vi "Execute.vi"(0 "reference in":refnum<class "ViPER.lvclass">, 1 "cmd":string, 2 "controls":string[](array[string]), 3 "indicators":string[](array[string]), 4 "control data":variant[](array[variant]), 5 "error in (no error)":errorcluster, 6 "must_exist":bool=TRUE, 7 "options":i32 format="%.0x", 9 "wait until done (T)":bool=TRUE) -> (14 "reference out":refnum<class "ViPER.lvclass">, 15 "exists":bool, 16 "vi reference":refnum<vi>, 18 "indicator data":variant[](array[variant]), 19 "error out":errorcluster)   [LabVIEW 2022 SP3, in "ViPER.lvlib" / "ViPER.lvclass"]
doc: "### BSD License (http://www.opensource.org/licenses/bsd-license.php) Begin ###\n\nCopyright (c) 2018 Kurt Friday www.medulla.net\n\nAll rights reserved.\n\nRedistribution and use in source and binary forms, with or without\nmodification, are permitted provided that the following conditions are met:\n\n * Redistributions of source code must retain the above copyright\n notice, this list of conditions and the following disclaimer.\n\n * Redistributions in binary form must reproduce the above copyright\n notice, this list of conditions and the following disclaimer in the\n documentation and/or other materials provided with the distribution.\n\n * Neither the name of the <organization> nor the\n names of its contributors may be used to endorse or promote products\n derived from this software without specific prior written permission.\n\nTHIS SOFTWARE IS PROVIDED BY THE COPYRIGHT HOLDERS AND CONTRIBUTORS \"AS IS\" AND\nANY EXPRESS OR IMPLIED WARRANTIES, INCLUDING, BUT NOT LIMITED TO, THE IMPLIED\nWARRANTIES OF MERCHANTABILITY AND FITNESS FOR A PARTICULAR PURPOSE ARE\nDISCLAIMED. IN NO EVENT SHALL <COPYRIGHT HOLDER> BE LIABLE FOR ANY\nDIRECT, INDIRECT, INCIDENTAL, SPECIAL, EXEMPLARY, OR CONSEQUENTIAL DAMAGES\n(INCLUDING, BUT NOT LIMITED TO, PROCUREMENT OF SUBSTITUTE GOODS OR SERVICES;\nLOSS OF USE, DATA, OR PROFITS; OR BUSINESS INTERRUPTION) HOWEVER CAUSED AND\nON ANY THEORY OF LIABILITY, WHETHER IN CONTRACT, STRICT LIABILITY, OR TORT\n(INCLUDING NEGLIGENCE OR OTHERWISE) ARISING IN ANY WAY OUT OF THE USE OF THIS\nSOFTWARE, EVEN IF ADVISED OF THE POSSIBILITY OF SUCH DAMAGE."
uses:
  ViPER.lvclass
panel:
  # "### BSD License (http://www.opensource.org/licenses/bsd-license.php) Begin ###\n\nCopyright (c) 2018  Kurt Friday www.medulla.net\n\nAll rights reserved.\n\nRedistribution and use in source and binary forms, with or without\nmodification, are permitted provided that the following conditions are met:\n\n    * Redistributions of source code must retain the above copyright\n      notice, this list of conditions and the following disclaimer.\n\n    * Redistributions in binary form must reproduce the above copyright\n      notice, this list of conditions and the following disclaimer in the\n      documentation and/or other materials provided with the distribution.\n\n    * Neither the name of the <organization> nor the\n      names of its contributors may be used to endorse or promote products\n      derived from this software without specific prior written permission.\n\nTHIS SOFTWARE IS PROVIDED BY THE COPYRIGHT HOLDERS AND CONTRIBUTORS \"AS IS\" AND\nANY EXPRESS OR IMPLIED WARRANTIES, INCLUDING, BUT NOT LIMITED TO, THE IMPLIED\nWARRANTIES OF MERCHANTABILITY AND FITNESS FOR A PARTICULAR PURPOSE ARE\nDISCLAIMED. IN NO EVENT SHALL <COPYRIGHT HOLDER> BE LIABLE FOR ANY\nDIRECT, INDIRECT, INCIDENTAL, SPECIAL, EXEMPLARY, OR CONSEQUENTIAL DAMAGES\n(INCLUDING, BUT NOT LIMITED TO, PROCUREMENT OF SUBSTITUTE GOODS OR SERVICES;\nLOSS OF USE, DATA, OR PROFITS; OR BUSINESS INTERRUPTION) HOWEVER CAUSED AND\nON ANY THEORY OF LIABILITY, WHETHER IN CONTRACT, STRICT LIABILITY, OR TORT\n(INCLUDING NEGLIGENCE OR OTHERWISE) ARISING IN ANY WAY OUT OF THE USE OF THIS\nSOFTWARE, EVEN IF ADVISED OF THE POSSIBILITY OF SUCH DAMAGE."
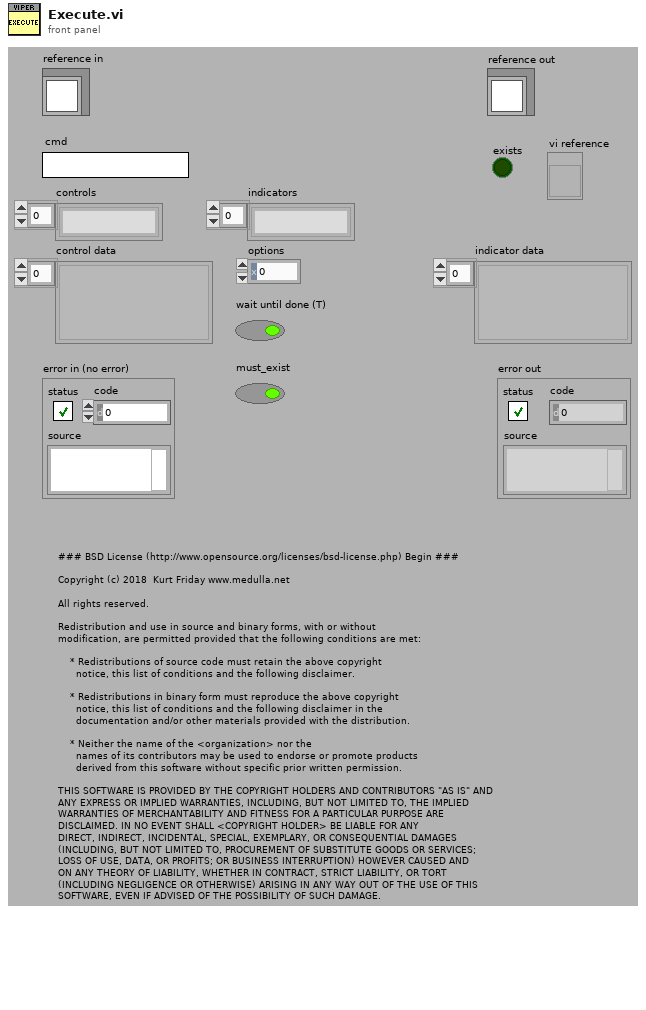
[diagram p1: front panel]
types:
  T1 = typedef "ViPER.lvlib/ViPER.lvclass/ObjectAttributes.ctl" = cluster{"Object":T2, "Ancestors":T4[], "Config":T5, "Init_OK":bool, "Hierachy":string[], "PPL?":bool[], "SFP_Open":bool[], "Config_SFP_Open":bool[], "SoftFP_event":refnum<user-event>[], "ConfigFP_event":refnum<user-event>[], "SoftFP_Shutdown_Notifier":refnum<notifier>[], "ConfigFP_Shutdown_Notifier":refnum<notifier>[]}
  T2 = typedef "ViPER.lvlib/ViPER.lvclass/ObjectDefinition.ctl" = cluster{"Name":string, "Ancestors":T3[]}
  T3 = typedef "ViPER.lvlib/ViPER.lvclass/Ancestor.ctl" = cluster{"Class":string, "Config":string, "Objects":string[]}
  T4 = typedef "ViPER.lvlib/ViPER.lvclass/ObjectLayers.ctl" = cluster{"Ancestor":string, "Objects":refnum<class "ViPER.lvclass">[], "Object_Names":string[], "Owned":bool[]}
  T5 = typedef "ViPER.lvlib/ViPER.lvclass/Config.ctl" = cluster{"default":string}
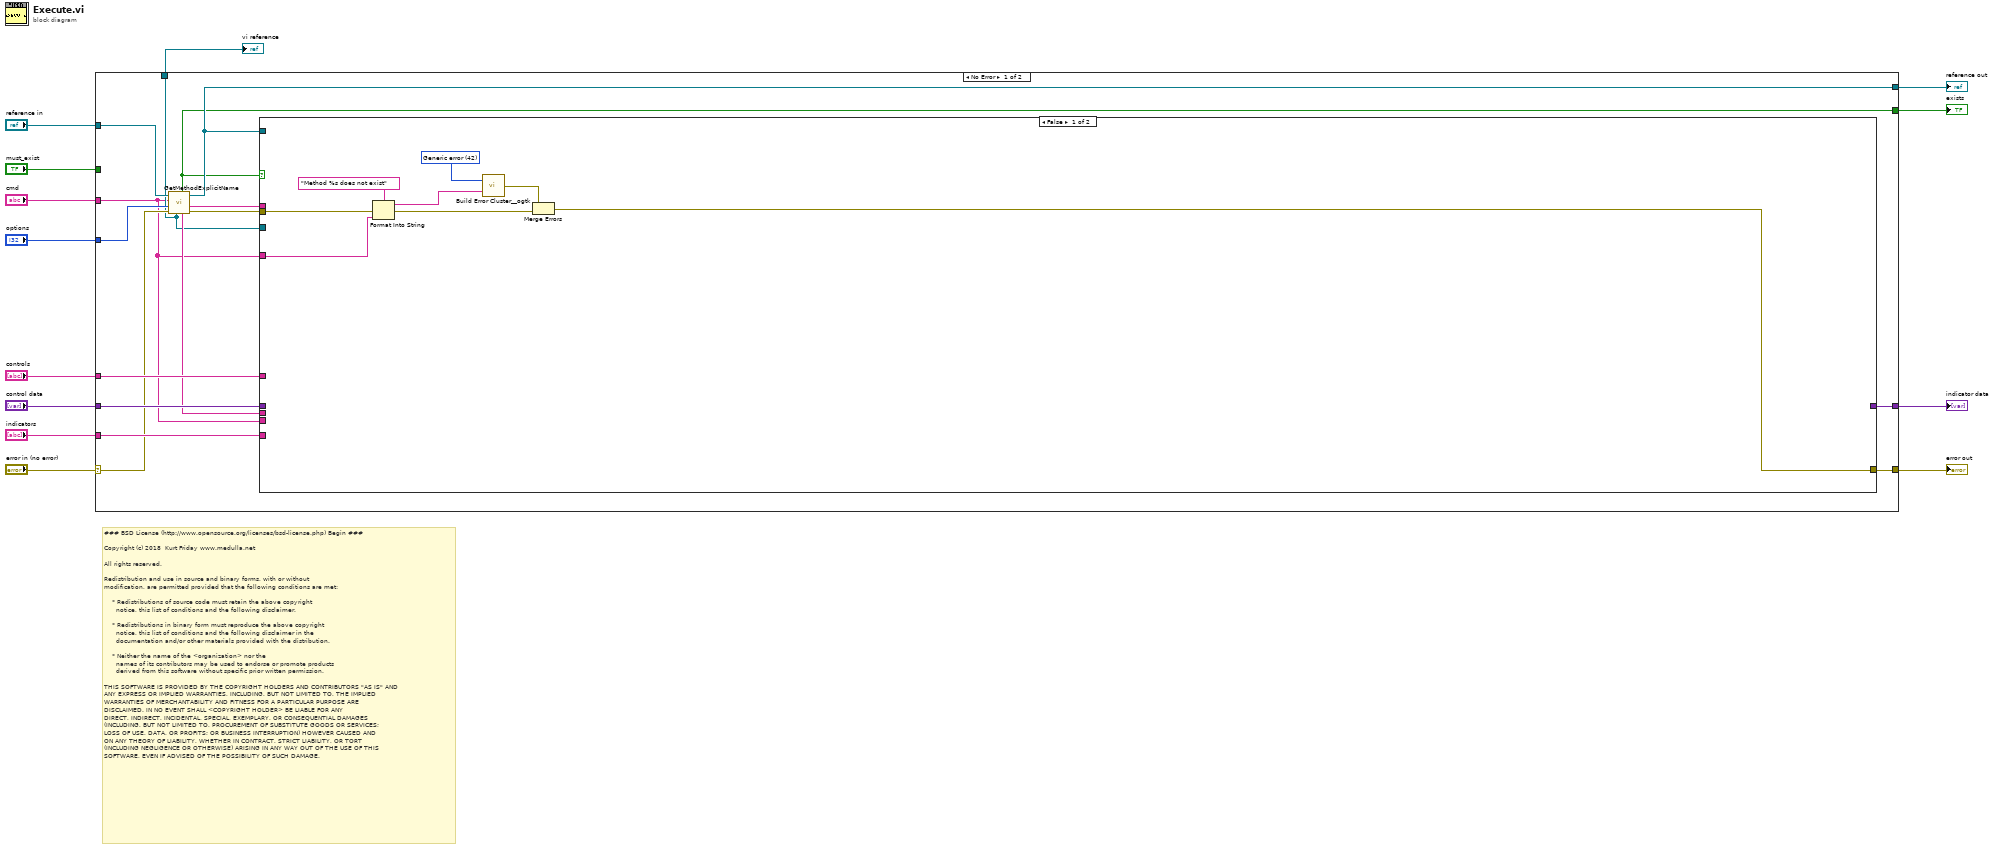
[diagram p0: block diagram]
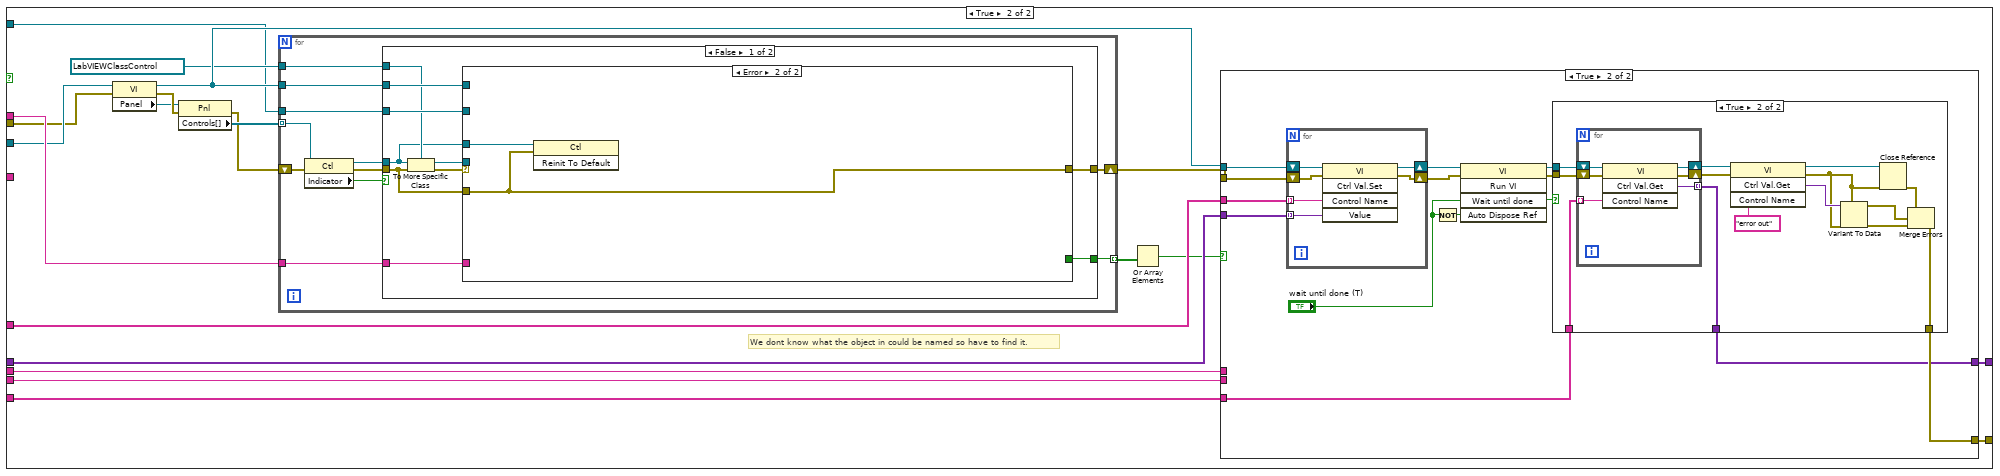
[diagram p2: hidden frame]
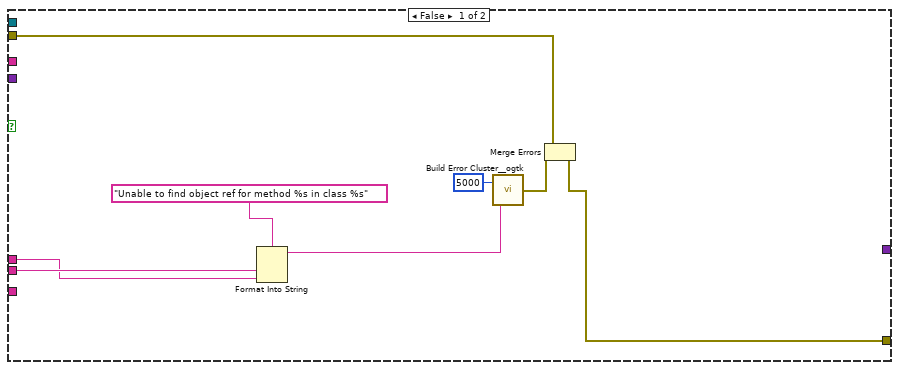
[diagram p3: hidden frame]
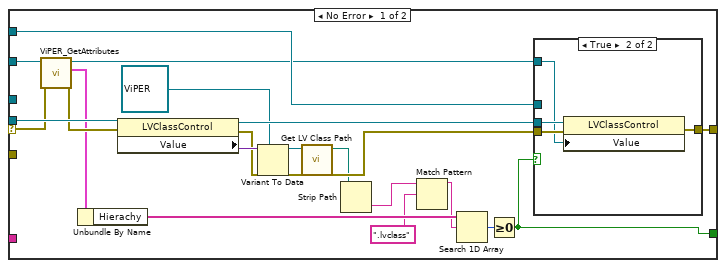
[diagram p5: hidden frame]
diagram:
  # "### BSD License (http://www.opensource.org/licenses/bsd-license.php) Begin ###\n\nCopyright (c) 2018  Kurt Friday www.medulla.net\n\nAll rights reserved.\n\nRedistribution and use in source and binary forms, with or without\nmodification, are permitted provided that the following conditions are met:\n\n    * Redistributions of source code must retain the above copyright\n      notice, this list of conditions and the following disclaimer.\n\n    * Redistributions in binary form must reproduce the above copyright\n      notice, this list of conditions and the following disclaimer in the\n      documentation and/or other materials provided with the distribution.\n\n    * Neither the name of the <organization> nor the\n      names of its contributors may be used to endorse or promote products\n      derived from this software without specific prior written permission.\n\nTHIS SOFTWARE IS PROVIDED BY THE COPYRIGHT HOLDERS AND CONTRIBUTORS \"AS IS\" AND\nANY EXPRESS OR IMPLIED WARRANTIES, INCLUDING, BUT NOT LIMITED TO, THE IMPLIED\nWARRANTIES OF MERCHANTABILITY AND FITNESS FOR A PARTICULAR PURPOSE ARE\nDISCLAIMED. IN NO EVENT SHALL <COPYRIGHT HOLDER> BE LIABLE FOR ANY\nDIRECT, INDIRECT, INCIDENTAL, SPECIAL, EXEMPLARY, OR CONSEQUENTIAL DAMAGES\n(INCLUDING, BUT NOT LIMITED TO, PROCUREMENT OF SUBSTITUTE GOODS OR SERVICES;\nLOSS OF USE, DATA, OR PROFITS; OR BUSINESS INTERRUPTION) HOWEVER CAUSED AND\nON ANY THEORY OF LIABILITY, WHETHER IN CONTRACT, STRICT LIABILITY, OR TORT\n(INCLUDING NEGLIGENCE OR OTHERWISE) ARISING IN ANY WAY OUT OF THE USE OF THIS\nSOFTWARE, EVEN IF ADVISED OF THE POSSIBILITY OF SUCH DAMAGE."
  n1 = case shown="No Error" "error in (no error)" {
    selector: "error in (no error)" -> [w21 w158]
    tunnel: [w28 w158] -> w12
    tunnel: [w19 w157] -> w10
    tunnel: "reference in" -> [w20 w157]
    tunnel: "cmd" -> [w14 _]
    tunnel: "control data" -> [w26 w156]
    tunnel: "controls" -> [w27 _]
    tunnel: "indicators" -> [w25 _]
    tunnel: [w24 w156] -> w5
    tunnel: "options" -> [w18 _]
    tunnel: "must_exist" -> [_ _]
    tunnel: [w15 _] -> w2
    tunnel: [w16 _] -> w1
    frame No Error {
      n2 = call "GetMethodExplicitName.vi"("error in (no error)"=w21, "options"=w18, "method"=w14, "Driver in"=w20) -> ("error out"=w17:errorcluster, "class explicit name"=w23:string, "Driver out"=w19:refnum<class "ViPER.lvclass">, "class"=w22:string, "exists"=w15:bool, "vi reference"=w16:refnum<vi>)  [unwired: 1 in, 1 out]
      n3 = case shown="False" w15 {
        tunnel: [w30 w56] -> w28
        tunnel: w27 -> [_ w55]
        tunnel: w26 -> [_ w54]
        tunnel: w25 -> [_ w53]
        tunnel: [_ w52] -> w24
        tunnel: w23 -> [_ w45]
        tunnel: w22 -> [_ w44]
        tunnel: w14 -> [_ w43]
        tunnel: w19 -> [_ w42]
        tunnel: w16 -> [_ w38]
        tunnel: w17 -> [w34 w37]
        tunnel: w14 -> [w35 _]
        frame False {
          w36 = 42 items=["No error", "Argument error", "Memory is full", "Out of zone", "End of file", "File already open", "Generic file I/O error", "File not found", "File permission error", "Disk is full", "Duplicate path", "Too many files open", "System feature not enabled", "Resource file not found", "Cannot add resource", "Resource not found", "Image not found", "Image memory error", "Pen does not exist", "Config type invalid", "Config token not found", "Config parse error", "Config memory error", "Bad external code format", "Bad external code offset", "External code not present", "Null window", "Destroy window error", "Null menu", "Print aborted", "Bad print record", "Print driver error", "Windows error during printing", "Memory error during printing", "Print dialog error", "Generic print error", "Invalid device refnum", "Device not found", "Device parameter error", "Device unit error", "Cannot open device", "Device call aborted", "Generic error", "Cancelled by user", "Object ID too low", "Object ID too high", "Object not in heap", "Unknown heap", "Unknown object (invalid DefProc)", "Unknown object (DefProc not in table)", "Message out of range", "Invalid (null) method", "Unknown message", "Manager call not supported", "Bad address", "Network operation in progress", "Network operation timed out", "Connection is busy", "Network attribute not supported", "Network error", "Address in use", "System out of memory", "Connection aborted", "Connection refused", "Not connected", "Already connected", "Connection closed", "Initialization error (interapplication manager)", "Bad occurrence", "Wait on unbound occurrence handler", "Occurrence queue overflow", "Datalog type conflict", "Unused", "Unrecognized type (interapplication manager)", "Memory corrupt", "Failed to make temporary DLL", "Old CIN version", "Drag socket not found", "Failed to load drop-object", "Failed to register OLE object", "Failed to release OLE object", "Format specifier type mismatch", "Unknown format specifier", "Too few format specifiers", "Too many format specifiers", "Scan failed", "Newer CIN version", "Error converting to variant", "Runtime menu error", "Password tampered", "Variant attribute not found", "Incompatible variant data type", "Event data is not available", "Event Store is not present", "Occurrence is not found", "Event Queue is not created", "Event info is not available", "Refnum passed is NULL", "Error retrieving Class GUID", "Error retrieving CoClass GUID", "Error retrieving TypeLib GUID.", "Bad built application magic bytes.", "Specific driver is different from the specific driver associated with the Logical Name.", "There is no session opened to the class driver.", "Max Error", "MAX - Error with config objects", "MAX - Error loading configuration", "MAX - Group not supported"]
          n4 = Format Into String(format string="Method %s does not exist", error in=w34, w35) -> (resulting string=w32:string, error out=w31:errorcluster)  [unwired: 1 in]
          n5 = call <userlib>:"Build Error Cluster__ogtk.vi"("String to Prepend to source (\"\")"=w32, "code"=w36) -> ("error out"=w29:errorcluster)
          n6 = Merge Errors(w29, w31) -> (w30:errorcluster)
        }
        frame True {
          # "We dont know what the object in could be named so have to find it."
          n7 = property class="VI"(reference=w38, error in=w37) -> (reference out=w49:refnum<vi>, error out=w51:errorcluster, "Panel"=w41:refnum<vi>)
          n8 = property class="Pnl"(reference=w41, error in=w51) -> (error out=w48:errorcluster, "Controls[]"=w50:refnum<vi>[])  [unwired: 1 out]
          n9 = for {
            tunnel: w50 -> [w105] mode=indexing
            tunnel: w45 -> [w112]
            tunnel: w42 -> [w110]
            tunnel: w49 -> [w111]
            shift-right: [w109] -> w47
            shift-left: w48 -> [w106]
            tunnel: [w108] -> w40 mode=indexing
            tunnel: refnum<vi> refnum ("reference in") -> [w107]
            n10 = property class="Ctl"(reference=w105, error in=w106) -> (reference out=w115:refnum<vi>, error out=w114:errorcluster, "Indicator"=w113:bool)
            n11 = case shown="False" w113 {
              tunnel: w115 -> [w116 _]
              tunnel: w114 -> [w117 w155]
              tunnel: w112 -> [w123 _]
              tunnel: [w122 _] -> w108
              tunnel: w111 -> [w121 _]
              tunnel: w110 -> [w120 _]
              tunnel: [w119 w155] -> w109
              tunnel: w107 -> [w118 _]
              frame False {
                n12 = To More Specific Class(target class=w118, reference=w116, error in=w117) -> (specific class reference=w125:refnum<vi>, error out=w124:errorcluster)
                n13 = case shown="Error" w124 {
                  selector: w124 -> [w134 _]
                  tunnel: w125 -> [w138 _]
                  tunnel: w123 -> [_ _]
                  tunnel: [w126 _] -> w122
                  tunnel: w121 -> [w146 _]
                  tunnel: w120 -> [w136 _]
                  tunnel: w117 -> [_ w153]
                  tunnel: [w145 w153] -> w119
                  tunnel: w116 -> [_ w154]
                  frame No Error {
                    n14 = call "ViPER_GetAttributes.vi"("error in (no error)"=w134, "reference in"=w136) -> ("error out"=w133:errorcluster, "Data"=w132:T1, "reference out"=w135:refnum<class "ViPER.lvclass">)  [unwired: 6 in, 1 out]
                    n15 = Unbundle By Name(w132) -> ("Hierachy"=w131:string[])
                    n16 = property class="LVClassControl"(reference=w138, error in=w133) -> (reference out=w147:refnum<vi>, error out=w141:errorcluster, "Value"=w142:variant)
                    n17 = Variant To Data(error in=w141, type=refnum<class "ViPER.lvclass"> refnum ("Driver in"), Variant=w142) -> (data=w139:refnum<class "ViPER.lvclass">, error out=w140:errorcluster)
                    n18 = call <vilib>:"Get LV Class Path.vi"("error in (no error)"=w140, "object"=w139) -> ("error out"=w144:errorcluster, "class path"=w143:path)  [unwired: 8 in]
                    n19 = Strip Path(path=w143) -> (name=w129:string)  [unwired: 1 out]
                    n20 = Match Pattern(string=w129, regular expression=".lvclass") -> (before substring=w128:string)  [unwired: 1 in, 3 out]
                    n21 = Search 1D Array(1D array=w131, element=w128) -> (index of element=w127:i32)  [unwired: 1 in]
                    n22 = Greater Or Equal To 0?(x=w127) -> (x >= 0?=w126:bool)
                    n23 = case shown="True" w126 {
                      tunnel: w147 -> [_ w152]
                      tunnel: w144 -> [w148 w151]
                      tunnel: w146 -> [_ _]
                      tunnel: w135 -> [_ w150]
                      tunnel: [w148 w149] -> w145
                      frame False {
                      }
                      frame True {
                        n24 = property class="LVClassControl"(reference=w152, error in=w151, "Value"=w150) -> (error out=w149:errorcluster)  [unwired: 1 out]
                      }
                    }
                  }
                  frame Error {
                    n25 = invoke class="Ctl" method="Reinit To Default"(reference=w154, error in=w153) -> ()  [unwired: 1 in, 3 out]
                  }
                }
              }
              frame True {
              }
            }
          }
          n26 = Or Array Elements(Boolean array=w40) -> (logical OR=w39:bool)
          n27 = case shown="True" w39 {
            tunnel: [w58 w73] -> w56
            tunnel: w55 -> [_ w72]
            tunnel: w54 -> [_ w71]
            tunnel: w53 -> [_ w70]
            tunnel: [_ w69] -> w52
            tunnel: w49 -> [_ w68]
            tunnel: w47 -> [w57 w67]
            tunnel: w43 -> [w63 _]
            tunnel: w44 -> [w62 _]
            frame False {
              n28 = Format Into String(format string="Unable to find object ref for method %s in class %s", w63, w62) -> (resulting string=w60:string)  [unwired: 2 in, 1 out]
              n29 = call <userlib>:"Build Error Cluster__ogtk.vi"("String to Prepend to source (\"\")"=w60, "code"=5000) -> ("error out"=w59:errorcluster)
              n30 = Merge Errors(w57, w59) -> (w58:errorcluster)
            }
            frame True {
              n31 = for {
                shift-right: [w101] -> w76
                shift-left: w67 -> [w103]
                shift-right: [w102] -> w77
                shift-left: w68 -> [w104]
                tunnel: w72 -> [w100] mode=indexing
                tunnel: w71 -> [w99] mode=indexing
                n32 = invoke class="VI" method="Ctrl Val.Set"(reference=w104, error in=w103, "Control Name"=w100, "Value"=w99) -> (reference out=w102:refnum<vi>, error out=w101:errorcluster)  [unwired: 1 in, 3 out]
              }
              n33 = Not(x="wait until done (T)") -> (.not. x?=w66:bool)
              n34 = invoke class="VI" method="Run VI"(reference=w77, error in=w76, "Wait until done"="wait until done (T)", "Auto Dispose Ref"=w66) -> (reference out=w75:refnum<vi>, error out=w74:errorcluster)  [unwired: 1 in, 3 out]
              n35 = case shown="True" "wait until done (T)" {
                tunnel: w75 -> [_ w92]
                tunnel: w74 -> [w78 w91]
                tunnel: [w78 w82] -> w73
                tunnel: w70 -> [_ w80]
                tunnel: [_ w79] -> w69
                frame False {
                }
                frame True {
                  n36 = for {
                    shift-right: [w96] -> w90
                    shift-left: w92 -> [w98]
                    shift-right: [w95] -> w87
                    shift-left: w91 -> [w97]
                    tunnel: w80 -> [w94] mode=indexing
                    tunnel: [w93] -> w79 mode=indexing
                    n37 = invoke class="VI" method="Ctrl Val.Get"(reference=w98, error in=w97, "Control Name"=w94) -> (reference out=w96:refnum<vi>, error out=w95:errorcluster, "Get Control Value Variant"=w93:variant)  [unwired: 1 in, 1 out]
                  }
                  n38 = invoke class="VI" method="Ctrl Val.Get"(reference=w90, error in=w87, "Control Name"="error out") -> (reference out=w89:refnum<vi>, error out=w83:errorcluster, "Get Control Value Variant"=w86:variant)  [unwired: 1 in, 1 out]
                  n39 = Variant To Data(error in=w83, type=w83, Variant=w86) -> (data=w84:errorcluster, error out=w85:errorcluster)
                  n40 = Close Reference(reference=w89, error in (no error)=w83) -> (error out=w81:errorcluster)
                  n41 = Merge Errors(w81, w84, w85) -> (w82:errorcluster)
                }
              }
            }
          }
        }
      }
    }
    frame Error {
    }
  }
  "error out" <- w12
  "reference out" <- w10
  "indicator data" <- w5
  "exists" <- w2
  "vi reference" <- w1
